vi "check if alarm name exists.vi"(10 "name to locate":string, 11 "alarms module configuration in":refnum<class "alarms module configuration.lvclass">) -> (0 "alarm config":T1, 1 "index":i32, 2 "found?":bool, 3 "alarms module configuration out":refnum<class "alarms module configuration.lvclass">)   [LabVIEW 2013, in "alarms module configuration.lvclass"]
uses:
  alarms module configuration.lvclass
  alarm configuration.ctl
  <vilib>/NI/Tag Bus Module Framework/channel/TBM channel.lvclass
  alarm comparison.ctl
  compare type.ctl
  boolean operation.ctl
  alarms module configuration.lvclass/alarms module configuration.ctl
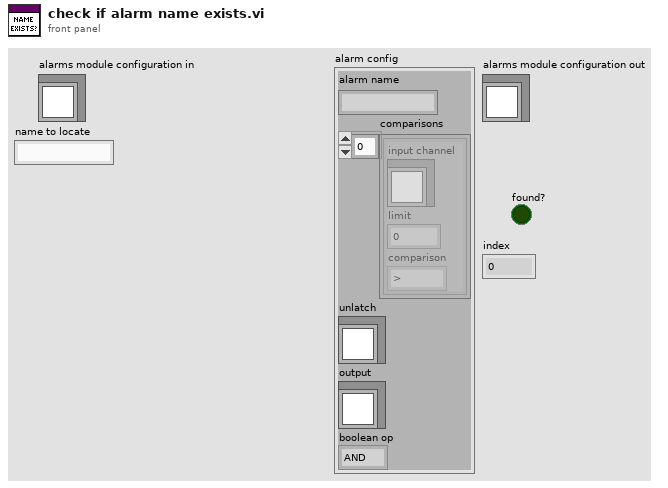
[diagram p1: front panel]
types:
  T1 = typedef "alarms module configuration.lvclass/alarm configuration.ctl" = cluster{"alarm name":string, "comparisons":T2[], "unlatch":refnum<class "TBM channel.lvclass">, "output":refnum<class "TBM channel.lvclass">, "boolean op":T4}
  T2 = typedef "alarms module configuration.lvclass/alarm comparison.ctl" = cluster{"input channel":refnum<class "TBM channel.lvclass">, "limit":dbl, "comparison":T3}
  T3 = typedef "alarms module configuration.lvclass/compare type.ctl" = enum16{">", "<", ">=", "<=", "="}
  T4 = typedef "alarms module configuration.lvclass/boolean operation.ctl" = enum16{"AND", "OR"}
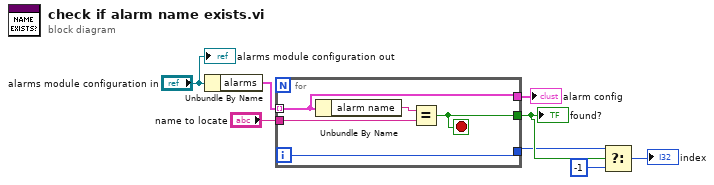
[diagram p0: block diagram]
diagram:
  n1 = Unbundle By Name("alarms module configuration in") -> ("alarms"=w7:T1[])
  n2 = for {
    tunnel: w7 -> [w9] mode=indexing
    tunnel: "name to locate" -> [w12]
    tunnel: [w11] -> w5
    tunnel: [w10] -> w4
    tunnel: [w9] -> w1
    i -> [w10]
    stop <- w11 stop-if-true
    n3 = Unbundle By Name(w9) -> ("alarm name"=w13:string)
    n4 = Equal?(x=w13, y=w12) -> (x = y?=w11:bool)
  }
  "found?" <- w5
  "alarm config" <- w1
  n5 = Select(t=w4, s=w5, f=-1) -> (s? t:f=→"index":i32)
  "alarms module configuration out" <- "alarms module configuration in"
